vi "Needs Grouping.vi"(7 "Pattern String Options":T1, 10 "Pattern Part":T2) -> (2 "Needs Grouping":bool)   [LabVIEW 2020, in "Stream.lvlib" / "URLPattern.lvclass"]
uses:
  URLPattern.lvclass
  Pattern Part.ctl
  Pattern Part Type.ctl
  Pattern Part Modifier.ctl
  Pattern String Options.ctl
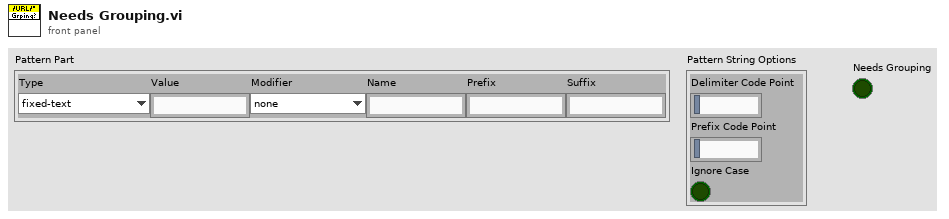
[diagram p1: front panel]
types:
  T1 = typedef "Stream.lvlib/URLPattern.lvclass/Pattern String Options.ctl" = cluster{"Delimiter Code Point":string, "Prefix Code Point":string, "Ignore Case":bool}
  T2 = typedef "Stream.lvlib/URLPattern.lvclass/Pattern Part.ctl" = cluster{"Type":T3, "Value":string, "Modifier":T4, "Name":string, "Prefix":string, "Suffix":string}
  T3 = typedef "Stream.lvlib/URLPattern.lvclass/Pattern Part Type.ctl" = enum16{"fixed-text", "regexp", "segment-wildcard", "full-wildcard"}
  T4 = typedef "Stream.lvlib/URLPattern.lvclass/Pattern Part Modifier.ctl" = enum16{"none", "optional", "zero-or-more", "one-or-more"}
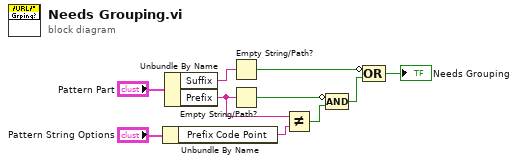
[diagram p0: block diagram]
diagram:
  n1 = Unbundle By Name("Pattern String Options") -> ("Prefix Code Point"=w5:string)
  n2 = Unbundle By Name("Pattern Part") -> ("Suffix"=w8:string, "Prefix"=w4:string)
  n3 = Empty String/Path?(string/path=w8) -> (empty?=w7:bool)
  n4 = Empty String/Path?(string/path=w4) -> (empty?=w3:bool)
  n5 = Not Equal?(x=w4, y=w5) -> (x != y?=w2:bool)
  n6 = Compound Arithmetic op=AND(invert w3, w2) -> (w1:bool)
  n7 = Compound Arithmetic op=OR(invert w7, w1) -> (→"Needs Grouping":bool)
